vi "Related To.vi"(11 "Relation in":refnum<class "Relation.lvclass">) -> (1 "error out":errorcluster, 2 "Related To":refnum<class "Entity.lvclass">)   [LabVIEW 2020, in "Conditum.lvlib" / "Columns.lvlib" / "Relation.lvclass"]
uses:
  Relation.lvclass
  Relation.lvclass/Relation.ctl
  Entity/Entity.lvclass
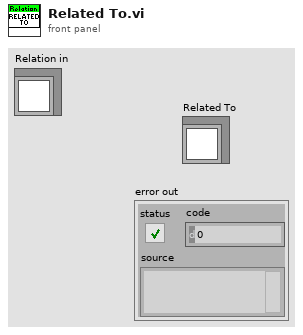
[diagram p1: front panel]
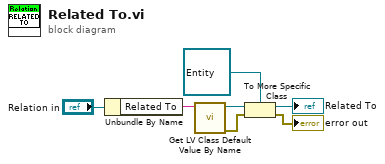
[diagram p0: block diagram]
diagram:
  n1 = Unbundle By Name("Relation in") -> ("Related To"=w6:string)
  n2 = call <vilib>:"Get LV Class Default Value By Name.vi"("class name"=w6) -> ("error out"=w2:errorcluster, "object"=w5:refnum<class>)  [unwired: 9 in]
  n3 = To More Specific Class(target class=refnum<class "Entity.lvclass"> refnum ("Conditum:Entity"), reference=w5, error in=w2) -> (specific class reference=→"Related To":refnum<class "Entity.lvclass">, error out=→"error out":errorcluster)
